vi "Write to Console.vi"(8 "error in (no error)":errorcluster caption="错误输入（无错误）", 11 "Input":string) -> (0 "error out":errorcluster caption="错误输出")   [LabVIEW 2015]
doc: "该模板用于创建子VI。"
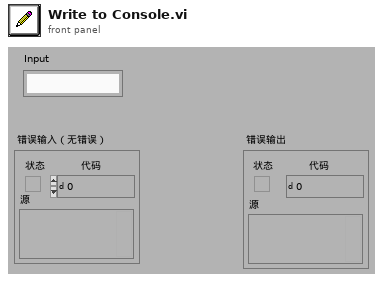
[diagram p1: front panel]
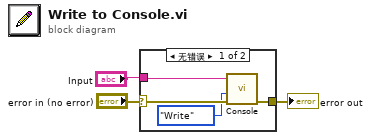
[diagram p0: block diagram]
diagram:
  n1 = case shown="无错误" "error in (no error)" {
    selector: "error in (no error)" -> [w7 w8]
    tunnel: [w6 w8] -> w2
    tunnel: "Input" -> [w4 _]
    frame No Error {
      n2 = call "Console.vi"("error in (no error)"=w7, "Mode"=enum16{"Write", "Read", "Clear"}."Write", "Input"=w4) -> ("error out"=w6:errorcluster)  [unwired: 7 in, 1 out]
    }
    frame Error {
    }
  }
  "error out" <- w2
